vi "_Axis_Stop.vi"(8 "Error In":errorcluster, 11 "轴序号":u16) -> (0 "Error Out":errorcluster)   [LabVIEW 2020, in "MT_API.lvlib"]
doc: "MT_API INT32 __stdcall MT_Set_Axis_Mode_Position_Close(WORD AObj);"
uses:
  MT_API.lvlib
  MT_API_64.dll
panel:
  out "函数返回值":i32
  # "关闭当前轴位置模式"
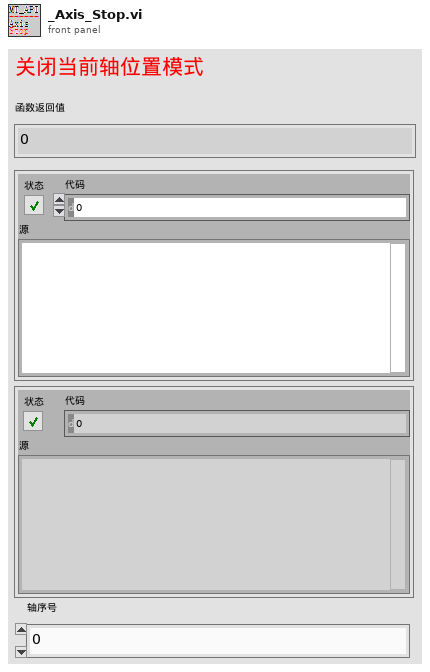
[diagram p1: front panel]
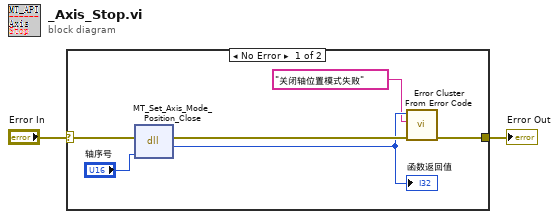
[diagram p0: block diagram]
diagram:
  n1 = case "条件结构" shown="No Error" "Error In" {
    selector: "Error In" -> [w7 w9]
    tunnel: [w4 w9] -> w1
    frame No Error {
      n2 = dll-call lib="D:/Project NJU/lib/MT/MT_API_64.*" fn="MT_Set_Axis_Mode_Position_Close"(error in=w7, "AObj"="轴序号") -> (error out=w6:errorcluster, "return type"=w5:i32)  [unwired: 3 in, 1 out]
      "函数返回值" <- w5
      n3 = call <vilib>:"Error Cluster From Error Code.vi"("error in (no error)"=w6, "error message (\"\")"="关闭轴位置模式失败", "error code (0)"=w5) -> ("error out"=w4:errorcluster)  [unwired: 6 in]
    }
    frame Error {
    }
  }
  "Error Out" <- w1
